vi "test.CreateDestroy.vi"() -> ()   [LabVIEW 2014]
uses:
  Private/Class/meth.Constructor.vi
  Private/Class/meth.Destructor.vi
  GLue.lvlib
panel:
  in  "Boolean":bool
  out "Numeric":i32
  out "error out":errorcluster
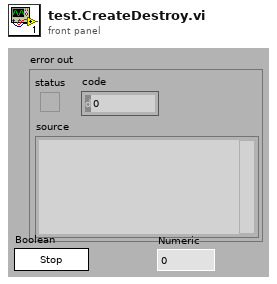
[diagram p1: front panel]
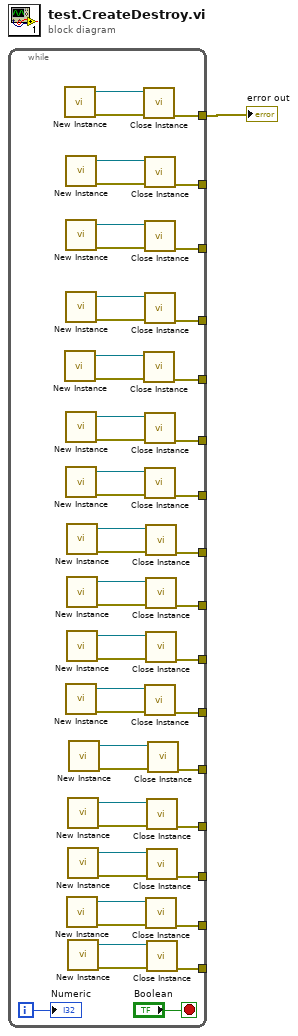
[diagram p0: block diagram]
diagram:
  n1 = while {
    tunnel: [w49] -> w1
    tunnel: [w40] -> _
    tunnel: [w39] -> _
    tunnel: [w38] -> _
    tunnel: [w37] -> _
    tunnel: [w32] -> _
    tunnel: [w31] -> _
    tunnel: [w26] -> _
    tunnel: [w25] -> _
    tunnel: [w20] -> _
    tunnel: [w19] -> _
    tunnel: [w14] -> _
    tunnel: [w13] -> _
    tunnel: [w8] -> _
    tunnel: [w7] -> _
    tunnel: [w2] -> _
    i -> [w48]
    stop <- "Boolean" stop-if-true
    n2 = call "New Instance.vi"() -> ("error out"=w50:errorcluster, "GLue out"=w51:refnum<class "class.GLue.lvclass">)  [unwired: 10 in]
    n3 = call "New Instance.vi"() -> ("error out"=w35:errorcluster, "GLue out"=w36:refnum<class "class.GLue.lvclass">)  [unwired: 10 in]
    n4 = call "New Instance.vi"() -> ("error out"=w46:errorcluster, "GLue out"=w45:refnum<class "class.GLue.lvclass">)  [unwired: 10 in]
    n5 = call "New Instance.vi"() -> ("error out"=w43:errorcluster, "GLue out"=w44:refnum<class "class.GLue.lvclass">)  [unwired: 10 in]
    n6 = call "New Instance.vi"() -> ("error out"=w42:errorcluster, "GLue out"=w41:refnum<class "class.GLue.lvclass">)  [unwired: 10 in]
    n7 = call "New Instance.vi"() -> ("error out"=w34:errorcluster, "GLue out"=w33:refnum<class "class.GLue.lvclass">)  [unwired: 10 in]
    n8 = call "New Instance.vi"() -> ("error out"=w29:errorcluster, "GLue out"=w30:refnum<class "class.GLue.lvclass">)  [unwired: 10 in]
    n9 = call "New Instance.vi"() -> ("error out"=w17:errorcluster, "GLue out"=w18:refnum<class "class.GLue.lvclass">)  [unwired: 10 in]
    n10 = call "New Instance.vi"() -> ("error out"=w28:errorcluster, "GLue out"=w27:refnum<class "class.GLue.lvclass">)  [unwired: 10 in]
    n11 = call "New Instance.vi"() -> ("error out"=w23:errorcluster, "GLue out"=w24:refnum<class "class.GLue.lvclass">)  [unwired: 10 in]
    n12 = call "New Instance.vi"() -> ("error out"=w22:errorcluster, "GLue out"=w21:refnum<class "class.GLue.lvclass">)  [unwired: 10 in]
    n13 = call "New Instance.vi"() -> ("error out"=w5:errorcluster, "GLue out"=w6:refnum<class "class.GLue.lvclass">)  [unwired: 10 in]
    n14 = call "New Instance.vi"() -> ("error out"=w11:errorcluster, "GLue out"=w12:refnum<class "class.GLue.lvclass">)  [unwired: 10 in]
    n15 = call "New Instance.vi"() -> ("error out"=w10:errorcluster, "GLue out"=w9:refnum<class "class.GLue.lvclass">)  [unwired: 10 in]
    n16 = call "New Instance.vi"() -> ("error out"=w4:errorcluster, "GLue out"=w3:refnum<class "class.GLue.lvclass">)  [unwired: 10 in]
    n17 = call "New Instance.vi"() -> ("error out"=w16:errorcluster, "GLue out"=w15:refnum<class "class.GLue.lvclass">)  [unwired: 10 in]
    n18 = call "Close Instance.vi"("error in"=w50, "GLue in"=w51) -> ("error out"=w49:errorcluster)  [unwired: 9 in]
    n19 = call "Close Instance.vi"("error in"=w35, "GLue in"=w36) -> ("error out"=w37:errorcluster)  [unwired: 9 in]
    n20 = call "Close Instance.vi"("error in"=w46, "GLue in"=w45) -> ("error out"=w40:errorcluster)  [unwired: 9 in]
    n21 = call "Close Instance.vi"("error in"=w43, "GLue in"=w44) -> ("error out"=w39:errorcluster)  [unwired: 9 in]
    n22 = call "Close Instance.vi"("error in"=w42, "GLue in"=w41) -> ("error out"=w38:errorcluster)  [unwired: 9 in]
    n23 = call "Close Instance.vi"("error in"=w34, "GLue in"=w33) -> ("error out"=w32:errorcluster)  [unwired: 9 in]
    n24 = call "Close Instance.vi"("error in"=w29, "GLue in"=w30) -> ("error out"=w31:errorcluster)  [unwired: 9 in]
    n25 = call "Close Instance.vi"("error in"=w17, "GLue in"=w18) -> ("error out"=w19:errorcluster)  [unwired: 9 in]
    n26 = call "Close Instance.vi"("error in"=w28, "GLue in"=w27) -> ("error out"=w26:errorcluster)  [unwired: 9 in]
    n27 = call "Close Instance.vi"("error in"=w23, "GLue in"=w24) -> ("error out"=w25:errorcluster)  [unwired: 9 in]
    n28 = call "Close Instance.vi"("error in"=w22, "GLue in"=w21) -> ("error out"=w20:errorcluster)  [unwired: 9 in]
    n29 = call "Close Instance.vi"("error in"=w5, "GLue in"=w6) -> ("error out"=w7:errorcluster)  [unwired: 9 in]
    n30 = call "Close Instance.vi"("error in"=w11, "GLue in"=w12) -> ("error out"=w13:errorcluster)  [unwired: 9 in]
    n31 = call "Close Instance.vi"("error in"=w10, "GLue in"=w9) -> ("error out"=w8:errorcluster)  [unwired: 9 in]
    n32 = call "Close Instance.vi"("error in"=w4, "GLue in"=w3) -> ("error out"=w2:errorcluster)  [unwired: 9 in]
    n33 = call "Close Instance.vi"("error in"=w16, "GLue in"=w15) -> ("error out"=w14:errorcluster)  [unwired: 9 in]
    "Numeric" <- w48
  }
  "error out" <- w1
